vi "G#Object_InstanceClassAttributes.vi"(0 "reference in":refnum<class "G#Object.lvclass">, 5 "error in (no error)":errorcluster) -> (14 "reference out":refnum<class "G#Object.lvclass">, 15 "static attribute ref":u32, 16 "created new?":bool, 19 "error out":errorcluster)   [LabVIEW 2020, in "G#Object.lvclass"]
doc: "Creates the object."
uses:
  G#Object.lvclass
  utils/G#Object_EventType.ctl
  utils/G#Object_ObjectInfoType.ctl
  utils/G#Object_CreateMethod.ctl
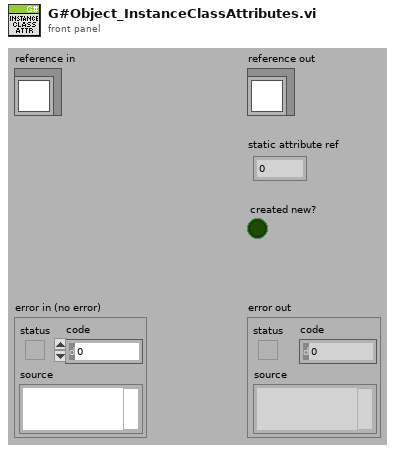
[diagram p1: front panel]
types:
  T1 = typedef "G#Object.lvclass/G#Object_ObjectInfoType.ctl" = cluster{"ObjectName":string, "ObjectID":u32, "Users":i32, "Counter":bool, "AttributeRefs":u32[], "FullClassName":string, "ClassName":string, "CreateMethod":T2, "GenericDestructorExists":bool, "Owner":string}
  T2 = typedef "G#Object.lvclass/G#Object_CreateMethod.ctl" = enum16{"Create", "Create or look up existing", "Look up existing"}
  T3 = typedef "G#Object.lvclass/G#Object_EventType.ctl" = enum16{"Created new", "Looked up existing", "Deleted", "Forced delete", "Not deleted", "Garbage collected", "Cleared", "User", "Error", "External create object", "External create class attributes", "Created class attributes", "Run constructor", "Run constructor done", "Run open method", "Run open method done"}
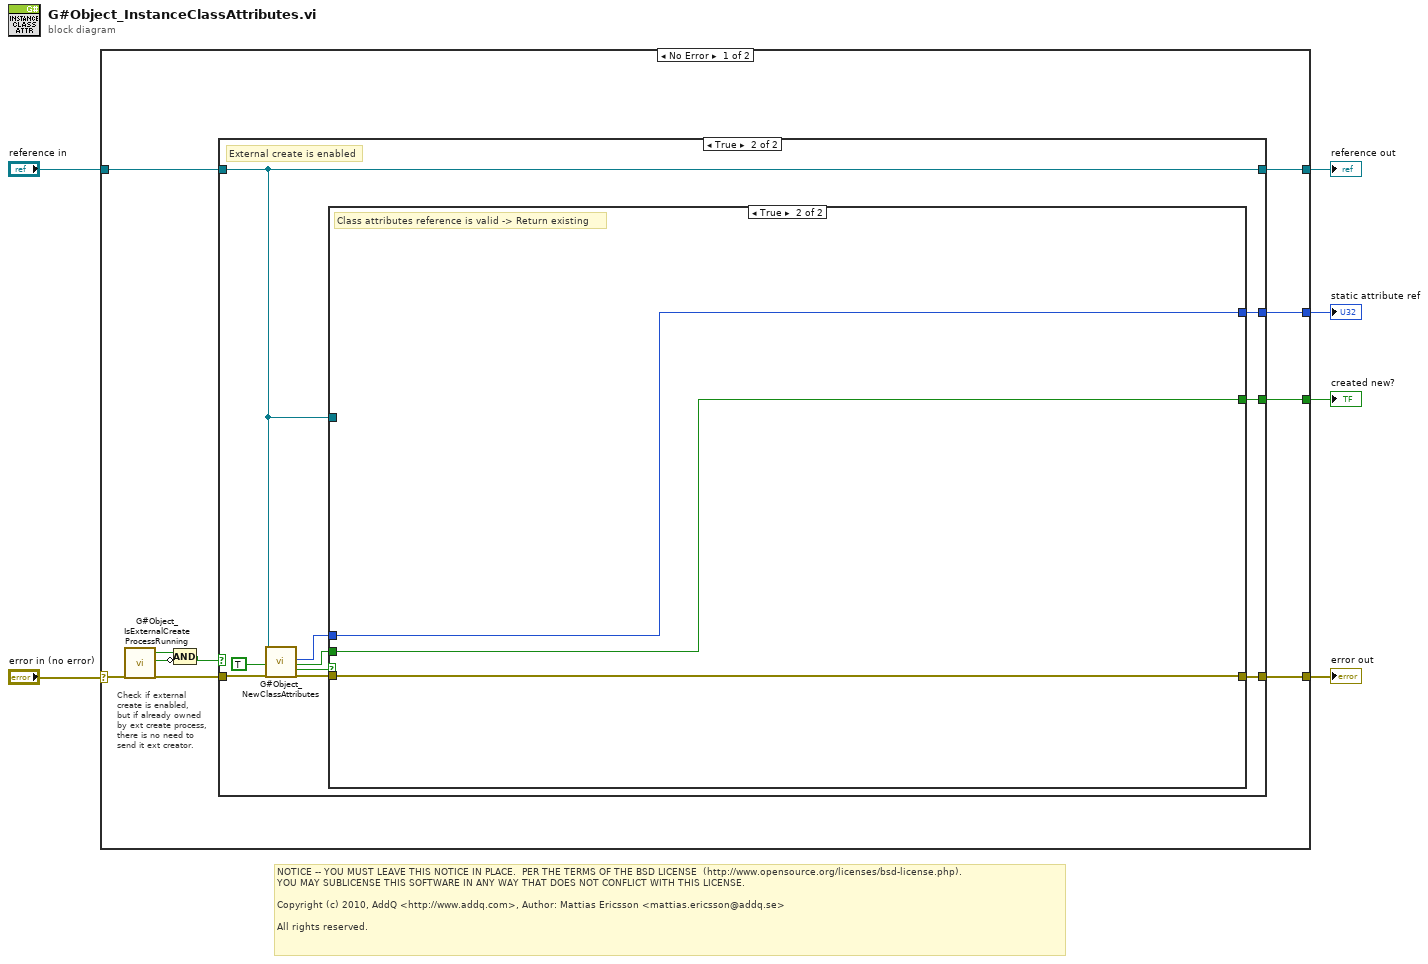
[diagram p0: block diagram]
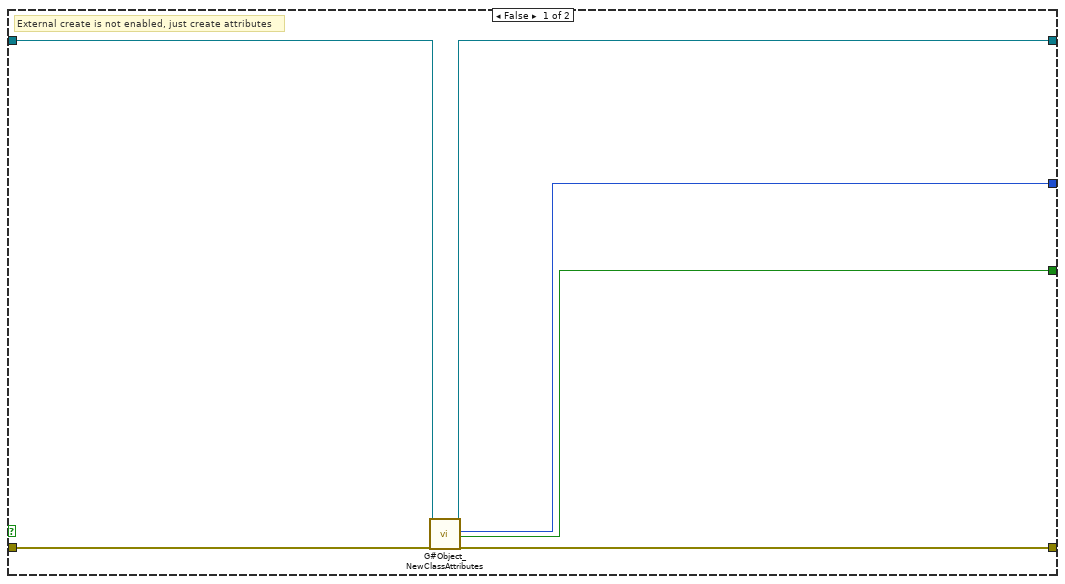
[diagram p2: hidden frame]
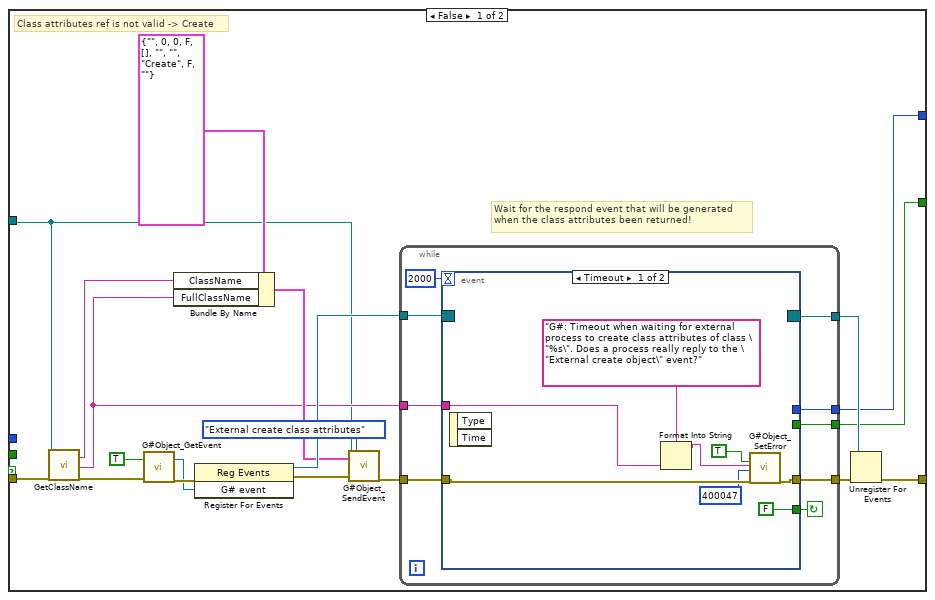
[diagram p3: hidden frame]
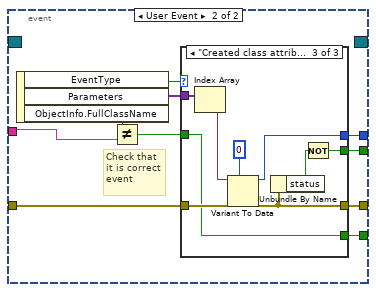
[diagram p4: hidden frame]
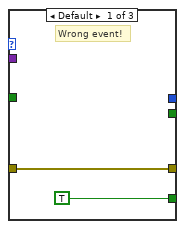
[diagram p5: hidden frame]
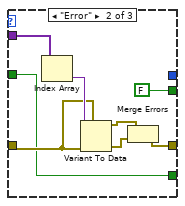
[diagram p6: hidden frame]
diagram:
  # "NOTICE -- YOU MUST LEAVE THIS NOTICE IN PLACE.  PER THE TERMS OF THE BSD LICENSE  (http://www.opensource.org/licenses/bsd-license.php).\nYOU MAY SUBLICENSE THIS SOFTWARE IN ANY WAY THAT DOES NOT CONFLICT WITH THIS LICENSE.\n\nCopyright (c) 2010, AddQ <http://www.addq.com>, Author: Mattias Ericsson <mattias.ericsson@addq.se>\n\nAll rights reserved."
  n1 = case shown="No Error" "error in (no error)" {
    selector: "error in (no error)" -> [w9 w102]
    tunnel: [w16 w102] -> w5
    tunnel: [w14 w101] -> w3
    tunnel: "reference in" -> [w15 w101]
    tunnel: [w13 _] -> w2
    tunnel: [w12 _] -> w1
    frame No Error {
      # "Check if external\ncreate is enabled,\nbut if already owned\nby ext create process,\nthere is no need to\nsend it ext creator."
      n2 = call "G#Object_IsExternalCreateProcessRunning.vi"("error in (no error)"=w9) -> ("external create enabled?"=w11:bool, "owned by external process?"=w10:bool, "error out"=w8:errorcluster)  [unwired: 15 in, 1 out]
      n3 = Compound Arithmetic op=AND(w11, invert w10) -> (w7:bool)
      n4 = case shown="True" w7 {
        tunnel: w8 -> [w22 w29]
        tunnel: [w21 w32] -> w16
        tunnel: w15 -> [w20 w27]
        tunnel: [w19 w27] -> w14
        tunnel: [w18 w31] -> w13
        tunnel: [w17 w30] -> w12
        frame False {
          # "External create is not enabled, just create attributes"
          n5 = call "G#Object_NewClassAttributes.vi"("reference in"=w20, "error in (no error)"=w22) -> ("reference out"=w19:refnum<class "G#Object.lvclass">, "static attribute ref"=w18:u32, "created new"=w17:bool, "error out"=w21:errorcluster)  [unwired: 13 in, 1 out]
        }
        frame True {
          # "External create is enabled"
          n6 = call "G#Object_NewClassAttributes.vi"("reference in"=w27, "check if valid only (F)"=TRUE ("check if valid only"), "error in (no error)"=w29) -> ("static attribute ref"=w25:u32, "created new"=w23:bool, "valid"=w24:bool, "error out"=w28:errorcluster)  [unwired: 12 in, 1 out]
          n7 = case shown="True" w24 {
            tunnel: [w42 w100] -> w32
            tunnel: [w38 w99] -> w31
            tunnel: [w36 w98] -> w30
            tunnel: w28 -> [w34 w100]
            tunnel: w27 -> [w33 _]
            tunnel: w25 -> [_ w99]
            tunnel: w23 -> [_ w98]
            frame False {
              # "Class attributes ref is not valid -> Create"
              # "Wait for the respond event that will be generated\nwhen the class attributes been returned!"
              n8 = call-dynamic "GetClassName.vi"("reference in"=w33, "error in (no error)"=w34) -> ("class name"=w40:string, "full class name"=w35:string, "error out"=w41:errorcluster)  [unwired: 13 in, 2 out]
              n9 = call "G#Object_GetEvent.vi"("create if needed (T)"=TRUE ("create if needed"), "error in (no error)"=w41) -> ("G# event"=w46:refnum<user-event>, "error out"=w49:errorcluster)  [unwired: 13 in, 3 out]
              n10 = Bundle By Name(cluster=T1 {"ObjectName"="", "ObjectID"=0, "Users"=0, "Counter"=FALSE, "AttributeRefs"=[], "FullClassName"="", "ClassName"="", "CreateMethod"=enum."Create", "GenericDestructorExists"=FALSE, "Owner"=""} ("ObjectInfo"), "ClassName"=w40, "FullClassName"=w35) -> (w37:T1)
              n11 = register-events(error in=w49, w46) -> (reference out=w45:refnum<event-registration>, error out=w48:errorcluster)  [unwired: 1 in]
              n12 = call "G#Object_SendEvent.vi"("reference in"=w33, "object info extended"=w37, "error in (no error)"=w48, "G# event type"=G#Object_EventType."External create class attributes") -> ("error out"=w47:errorcluster)  [unwired: 15 in]
              n13 = while {
                tunnel: w47 -> [w60]
                tunnel: w45 -> [w59]
                tunnel: [w58] -> w44
                tunnel: [w57] -> w43
                tunnel: [w54] -> w38
                tunnel: [w53] -> w36
                tunnel: w35 -> [w52]
                stop <- w56 continue-if-true
                n14 = event shown="[0] Timeout" {
                  selector: w59 -> [_ _]
                  dyn-events: [_ _] -> w58
                  timeout: 2000 -> [_ _]
                  tunnel: w60 -> [w67 w78]
                  tunnel: [w68 w77] -> w57
                  tunnel: [FALSE w76] -> w56
                  tunnel: [_ w73] -> w54
                  tunnel: [_ w72] -> w53
                  tunnel: w52 -> [w63 w70]
                  event Timeout {
                    n15 = event-data() -> ()  [unwired: 1 in, 2 out]
                    n16 = Format Into String(format string="G#: Timeout when waiting for external process to create class attributes of class \"%s\". Does a process really reply to the \"External create object\" event?", w63) -> (resulting string=w64:string)  [unwired: 2 in, 1 out]
                    n17 = call "G#Object_SetError.vi"("error (F)"=TRUE ("error"), "source"=w64, "code"=400047, "error in (no error)"=w67) -> ("error out"=w68:errorcluster)  [unwired: 15 in]
                  }
                  event User Event {
                    # "Check that\nit is correct\nevent"
                    n18 = event-data() -> ("EventType"=w75:T3, "Parameters"=w74:variant[], "ObjectInfo.FullClassName"=w71:string)  [unwired: 1 in]
                    n19 = Not Equal?(x=w71, y=w70) -> (x != y?=w69:bool)
                    n20 = case shown="\"Created class attributes\"" w75 {
                      tunnel: w78 -> [w80 w86 w96]
                      tunnel: [w80 w85 w90] -> w77
                      tunnel: [TRUE w81 w92] -> w76
                      tunnel: w74 -> [_ w88 w97]
                      tunnel: [_ _ w93] -> w73
                      tunnel: w69 -> [_ w81 w92]
                      tunnel: [_ FALSE w89] -> w72
                      frame Default {
                        # "Wrong event!"
                      }
                      frame "Error" {
                        n21 = Index Array(array=w88) -> (element=w87:variant)  [unwired: 1 in]
                        n22 = Variant To Data(error in=w86, type=w86, Variant=w87) -> (data=w84:errorcluster, error out=w83:errorcluster)
                        n23 = Merge Errors(w84, w83) -> (w85:errorcluster)
                      }
                      frame "Created class attributes" {
                        n24 = Index Array(array=w97) -> (element=w94:variant)  [unwired: 1 in]
                        n25 = Variant To Data(error in=w96, type=u32 0 ("static attribute ref"), Variant=w94) -> (data=w93:u32, error out=w90:errorcluster)
                        n26 = Unbundle By Name(w90) -> ("status"=w91:bool)
                        n27 = Not(x=w91) -> (.not. x?=w89:bool)
                      }
                    }
                  }
                }
              }
              n28 = Unregister For Events(event registration refnum=w44, error in=w43) -> (error out=w42:errorcluster)
            }
            frame True {
              # "Class attributes reference is valid -> Return existing"
            }
          }
        }
      }
    }
    frame Error {
    }
  }
  "error out" <- w5
  "reference out" <- w3
  "static attribute ref" <- w2
  "created new?" <- w1
